vi "UnregisterPublisher.vi"(7 "Topic Name":string, 8 "error in (no error)":errorcluster, 11 "Message Broker Interface TAP in":refnum<class "Message Broker Interface Ref.lvclass">) -> (0 "error out":errorcluster, 3 "Message Broker Interface TAP out":refnum<class "Message Broker Interface Ref.lvclass">)   [LabVIEW 2016, in "Stream Mediator.lvlib" / "Message Broker Interface Ref.lvclass"]
doc: "--\nCopyright © 2017 Composed SystemsI All rights reserved.\n\nAuthor: Jon McBee <jon.mcbee@composed.io>\n\nThis library is provided \"AS IS\" ,WITHOUT WARRANTIES OR\nCONDITIONS OF ANY KIND, either express or implied.\n\nComposed Systems -- composed.io\n\nStream 0.0.1.1\nJon McBee - Composed Systems\nCopyright (c) 2017, Composed Systems"
uses:
  <userlib>/Composed Systems/Stream/Mediator/Classes/Message Broker Interface Ref/Message Broker Interface Ref.lvclass
  <userlib>/Composed Systems/Stream/Mediator/Classes/Message Broker Interface Ref/Message Broker Interface Ref.lvclass/Message Broker Interface Ref.ctl
  <userlib>/Composed Systems/Stream/Mediator/Classes/Message Broker/Message Broker.lvclass
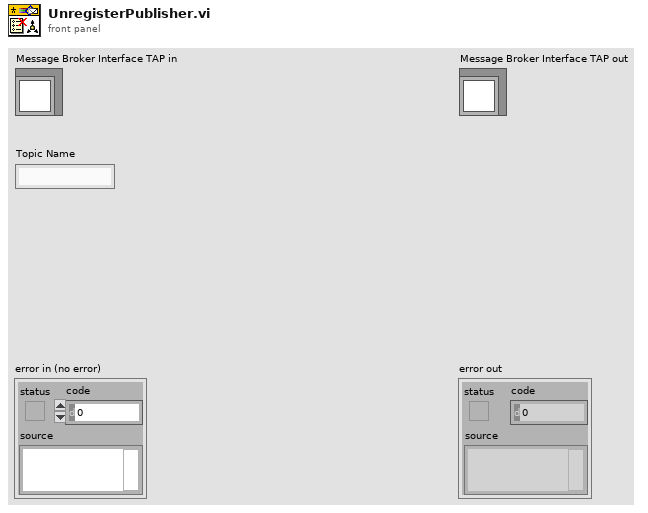
[diagram p1: front panel]
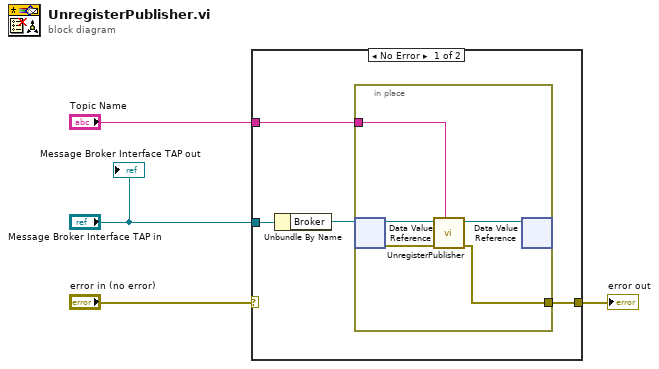
[diagram p0: block diagram]
diagram:
  n1 = case shown="No Error" "error in (no error)" {
    selector: "error in (no error)" -> [_ w14]
    tunnel: "Message Broker Interface TAP in" -> [w8 _]
    tunnel: [w5 w14] -> w2
    tunnel: "Topic Name" -> [w6 _]
    frame No Error {
      n2 = Unbundle By Name(w8) -> ("Broker"=w7:refnum<data-value>)
      n3 = in-place {
        in-place-border: w6 -> [w11]
        in-place-border: [w9] -> w5
        n4 = in-place-dvr #1(w7) -> (w13:refnum<class "Message Broker.lvclass">, w10:errorcluster)
        n5 = call <userlib>:"UnregisterPublisher.vi"("Topic Name"=w11, "error in (no error)"=w10, "Message Broker in"=w13) -> ("error out"=w9:errorcluster, "Message Broker out"=w12:refnum<class "Message Broker.lvclass">)  [unwired: 7 in]
        n6 = in-place-dvr #1(w12) -> ()  [unwired: 2 out]
      }
    }
    frame Error {
    }
  }
  "error out" <- w2
  "Message Broker Interface TAP out" <- "Message Broker Interface TAP in"
